vi "GetSwerveAbsoluteAzimuth.vi"(0 "Relative Position (Raw Sensor Units)":dbl) -> (1 "Azimuth Position (deg) [-180,+180]":dbl, 2 "Current Unwrapped Angle (deg) [-Inf,+Inf]":dbl)   [LabVIEW 2023]
doc: "Converts the relative azimuth encoder reading to an absolute azimuth angle."
uses:
  GlobalDrivebase.vi
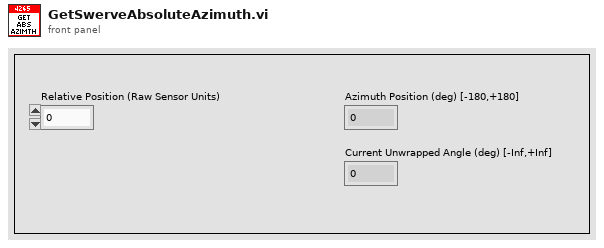
[diagram p1: front panel]
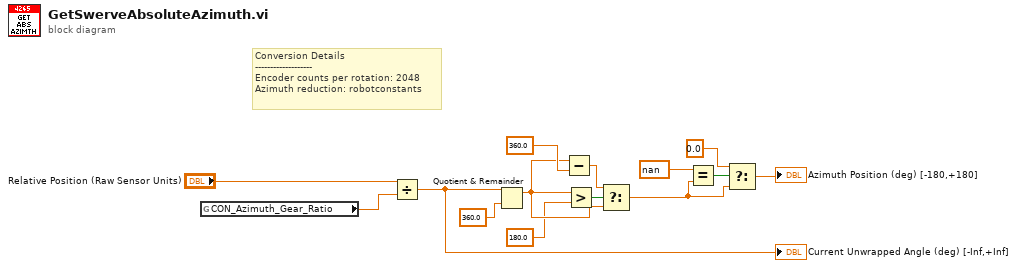
[diagram p0: block diagram]
diagram:
  # "Conversion Details\n-------------------\nEncoder counts per rotation: 2048\nAzimuth reduction: robotconstants"
  n1 = global read "GlobalDrivebase.vi" "CON_Azimuth_Gear_Ratio"() -> (w1:dbl)
  n2 = Divide(x="Relative Position (Raw Sensor Units)", y=w1) -> (x/y=w2:dbl)
  "Current Unwrapped Angle (deg) [-Inf,+Inf]" <- w2
  n3 = Quotient & Remainder(x=w2, y=360.0) -> (x-y*floor(x/y)=w11:dbl)  [unwired: 1 out]
  n4 = Subtract(x=w11, y=360.0) -> (x-y=w12:dbl)
  n5 = Greater?(x=w11, y=180.0) -> (0:w10:bool)
  n6 = Select(t=w12, s=w10, f=w11) -> (s? t:f=w5:dbl)
  n7 = Equal?(x=nan, y=w5) -> (x = y?=w6:bool)
  n8 = Select(t=0.0, s=w6, f=w5) -> (s? t:f=→"Azimuth Position (deg) [-180,+180]":dbl)
